vi "条件探针.vi"() -> ()   [LabVIEW 2021]
doc: "本VI是为《我和LabVIEW》一书编写的示例。\n关于本书的介绍请参考网页：\nhttp://ruanqizhen.spaces.live.com/blog/cns!5852D4F797C53FB6!4310.entry"
panel:
  out "y":dbl
  in  "x":dbl
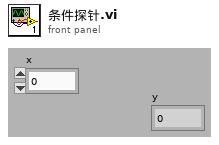
[diagram p1: front panel]
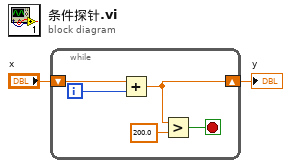
[diagram p0: block diagram]
diagram:
  n1 = while {
    shift-right: [w5] -> w1
    shift-left: "x" -> [w7]
    i -> [w6]
    stop <- w3 stop-if-true
    n2 = Add(x=w7, y=w6) -> (x+y=w5:dbl)
    n3 = Greater?(x=w5, y=200.0) -> (0:w3:bool)
  }
  "y" <- w1
